vi "Configure Gated Mode.vi"(0 "VISA resource name":refnum<visa-resource-name>, 1 "Channel (1:Channel 1)":i32(ring)=1 items=["Channel 1"=1, "Channel 2"=2], 2 "Gated Period (0.01 s)":dbl=0.01, 5 "Enable Gated Mode (T:Enable)":bool=TRUE, 7 "Trigger Source (0: Internal)":u16(ring) items=["Internal", "External"], 9 "Start Phase (0.0 degrees)":dbl=0.002 min=0.0 max=360.0 format="%#.1g", 11 "error in (no error)":errorcluster, 12 "Gate Polarity (0: Positive)":u16(ring) items=["Positive", "Negative"]) -> (4 "VISA resource name out":refnum<visa-resource-name>, 15 "error out":errorcluster)   [LabVIEW 2023, in "Siglent SDG X Series.lvlib"]
doc: "Configures and enables gated output mode."
uses:
  Siglent SDG X Series.lvlib
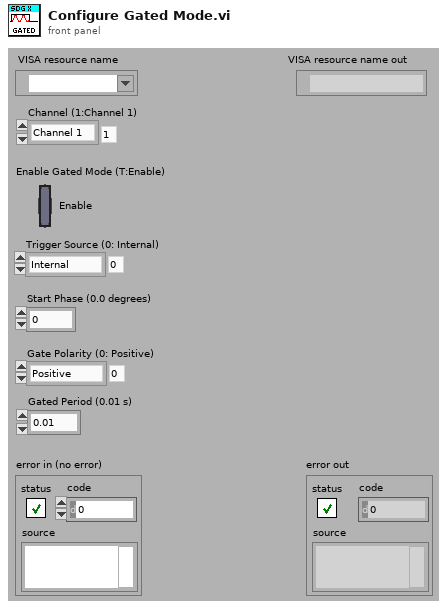
[diagram p1: front panel]
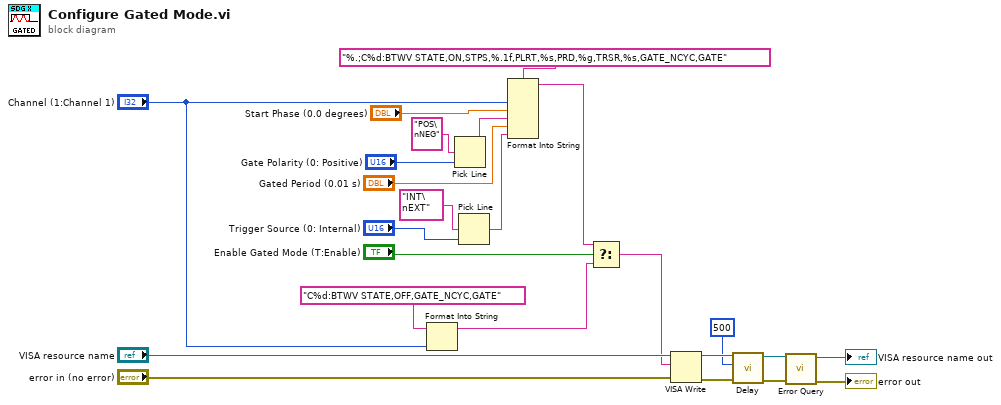
[diagram p0: block diagram]
diagram:
  n1 = Format Into String(format string="C%d:BTWV STATE,OFF,GATE_NCYC,GATE", "Channel (1:Channel 1)") -> (resulting string=w13:string)  [unwired: 2 in, 1 out]
  n2 = Pick Line(multi-line string="POS\nNEG", line index="Gate Polarity (0: Positive)") -> (output string=w16:string)  [unwired: 1 in]
  n3 = Pick Line(multi-line string="INT\nEXT", line index="Trigger Source (0: Internal)") -> (output string=w2:string)  [unwired: 1 in]
  n4 = Format Into String(format string="%.;C%d:BTWV STATE,ON,STPS,%.1f,PLRT,%s,PRD,%g,TRSR,%s,GATE_NCYC,GATE", "Channel (1:Channel 1)", "Start Phase (0.0 degrees)", w16, "Gated Period (0.01 s)", w2) -> (resulting string=w12:string)  [unwired: 2 in, 1 out]
  n5 = Select(t=w12, s="Enable Gated Mode (T:Enable)", f=w13) -> (s? t:f=w11:string)
  n6 = VISA Write(VISA resource name="VISA resource name", write buffer=w11, error in (no error)="error in (no error)") -> (VISA resource name out=w24:refnum<visa-resource-name>, error out=w23:errorcluster)  [unwired: 1 out]
  n7 = call "Delay.vi"("error in (no error)"=w23, "Delay Time (10)"=u32 500, "VISA resource name"=w24) -> ("error out"=w8:errorcluster, "VISA resource name out"=w7:refnum<visa-resource-name>)  [unwired: 7 in]
  n8 = call "Error Query.vi"("error in (no error)"=w8, "VISA resource name"=w7) -> ("error out"=→"error out":errorcluster, "VISA resource name out"=→"VISA resource name out":refnum<visa-resource-name>)  [unwired: 6 in, 2 out]
